vi "Init DB-SQLite.vi"(6 "File Option":T1(ring), 7 "DLL-Filepath":path, 8 "error in":errorcluster, 9 "busy timeout (ms)":i32=5000, 10 "DB-Filepath":string, 11 "DB-SQLite in":refnum<class "DB-SQLite.lvclass">) -> (0 "error out":errorcluster, 3 "DB-SQLite out":refnum<class "DB-SQLite.lvclass">)   [LabVIEW 2022 SP3, in "hse-db-sqlite.lvlib" / "DB-SQLite.lvclass"]
doc: "____\nHAMPEL SOFTWARE ENGINEERING v1.4.0 (2023-12-19 09:52)"
uses:
  DB-SQLite.lvclass
  DB-SQLite.lvclass/DB-SQLite.ctl
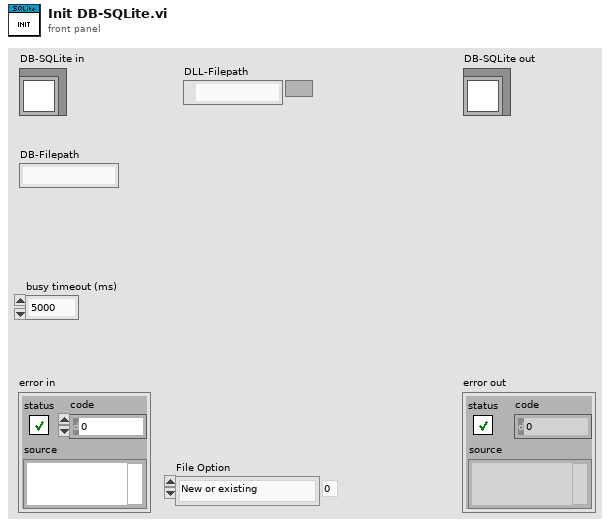
[diagram p1: front panel]
types:
  T1 = enum16{"New or existing", "Existing", "Read only"}
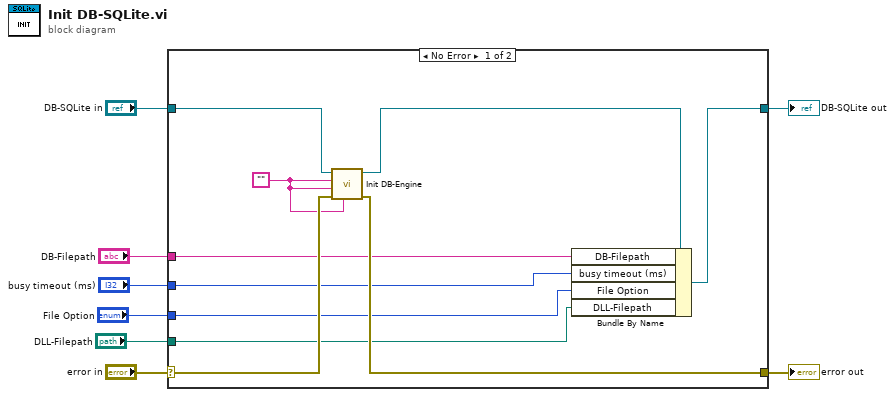
[diagram p0: block diagram]
diagram:
  n1 = case shown="No Error" "error in" {
    selector: "error in" -> [w17 w20]
    tunnel: [w16 w20] -> w7
    tunnel: [w13 w19] -> w5
    tunnel: "DB-SQLite in" -> [w18 w19]
    tunnel: "DB-Filepath" -> [w9 _]
    tunnel: "File Option" -> [w11 _]
    tunnel: "busy timeout (ms)" -> [w12 _]
    tunnel: "DLL-Filepath" -> [w10 _]
    frame No Error {
      w15 = ""
      n2 = call-dynamic "Init DB-Engine.vi"("Database"=w15, "error in"=w17, "Password"=w15, "User"=w15, "DB-Engine in"=w18) -> ("error out"=w16:errorcluster, "DB-Engine out"=w14:refnum<class "DB-SQLite.lvclass">)  [unwired: 5 in]
      n3 = Bundle By Name(cluster=w14, "DB-Filepath"=w9, "busy timeout (ms)"=w12, "File Option"=w11, "DLL-Filepath"=w10) -> (w13:refnum<class "DB-SQLite.lvclass">)
    }
    frame Error {
    }
  }
  "error out" <- w7
  "DB-SQLite out" <- w5
